vi "Inverse Kinematics.vi"() -> ()   [LabVIEW 2018]
uses:
  <vilib>/Platform/TimedLoop/XDataNode/timing_clust.ctl
  <vilib>/Platform/TimedLoop/XDataNode/nitl_modes.ctl
  <vilib>/Platform/TimedLoop/XDataNode/wakeup.ctl
  <extravilib>/ChannelInstances/Tag-bool/Read With Abort.vi
  <extravilib>/ChannelInstances/Tag-bool/Write With Abort.vi
  <extravilib>/ChannelInstances/Tag-bool/Instantiate.vi
  <extravilib>/ChannelInstances/Tag-bool/EndpointRead.vi
  <extravilib>/ChannelInstances/Tag-bool/Endpoint.vi
  <vilib>/Platform/TimedLoop/XDataNode/XDataNode.xnode
  <vilib>/Platform/TimedLoop/XDataNode/XDNodeRunTimeDep.lvlib
  <extravilib>/ChannelInstances/Tag-bool.lvlib
panel:
  out "Camera Image":T1(plugin-control)
  in  "Stop Button":bool
  out "Calibrated":bool
  out "Actual Joint \nCoordinates (rad)":dbl[](array[numeric])
  out "Joint Coordinates \nfrom Inv Kin (rad)":dbl[](array[numeric])
  in  "Task Coordinates for\nInv Kin (cm)":dbl[](array[numeric])=[3.81, 10.0]
  out "Motor angles (rad)":T2(graph)
  # "Mechatronic Systems Board"
  # "Inverse Kinematics"
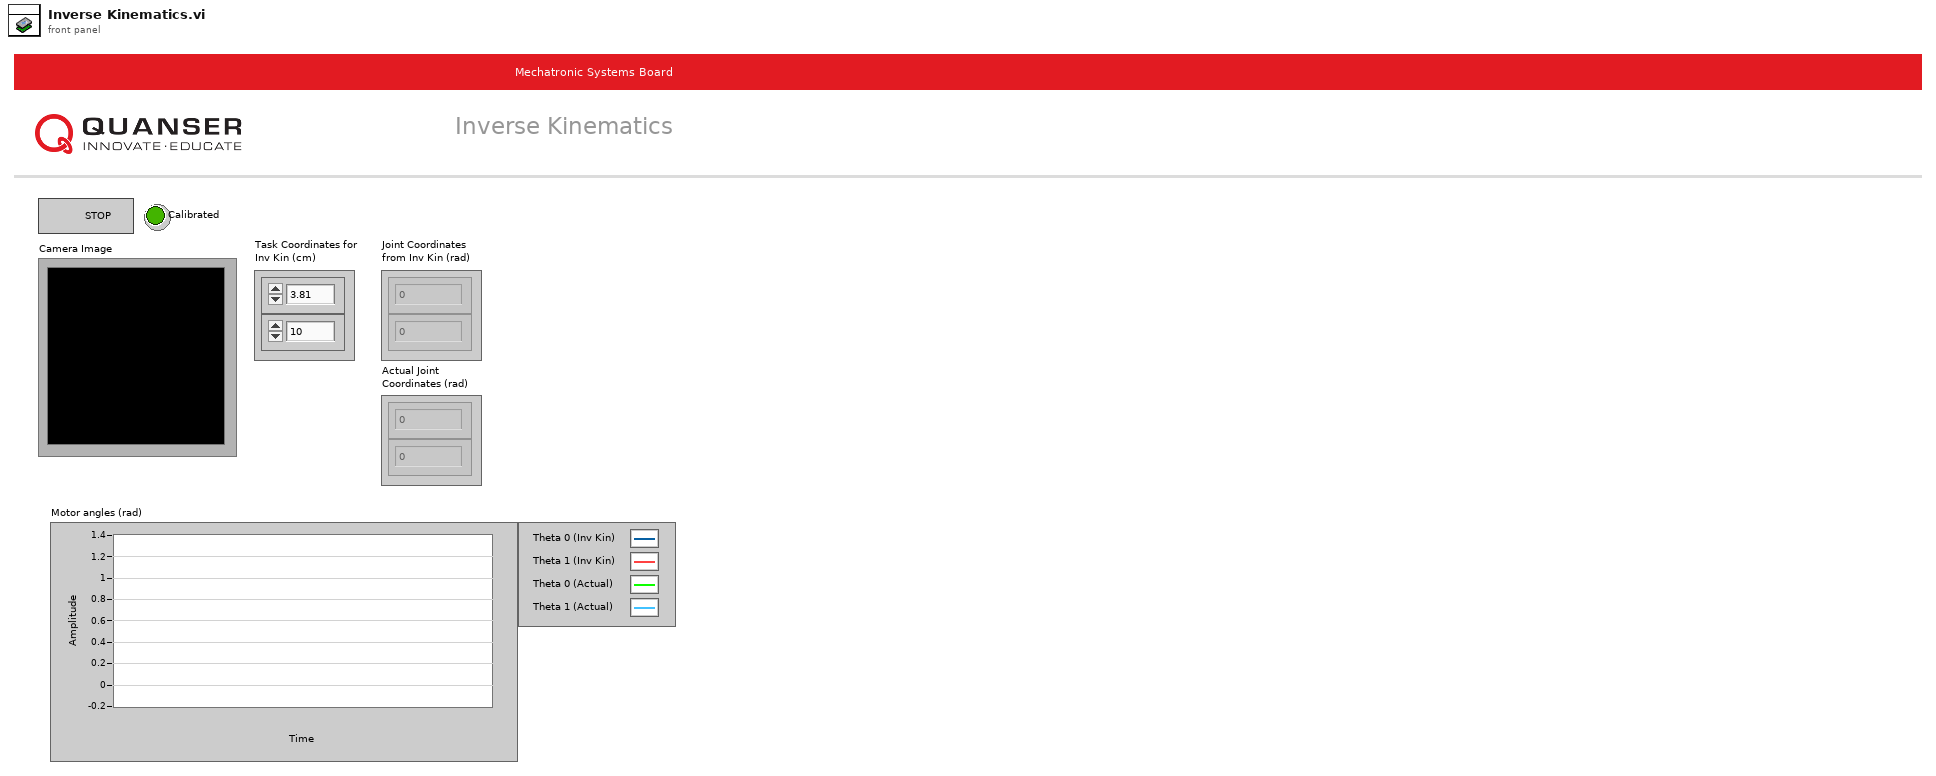
[diagram p1: front panel]
types:
  T1 = typedef "IMAQ Image.ctl" = refnum<image>
  T2 = cluster{dbl, dbl, "Numeric Control":dbl, "Numeric Control":dbl}
  T3 = typedef "QNET MS IO Cluster.ctl" = cluster{"Error":errorcluster, "Encoder Calibration Values":i32[], "Update Calibration":bool, "JPEG Resolutions":u16, "Raw Resolutions":u16, "Image Mode":enum16{"RAW RGB", "RAW Gray Scale", "JPEG"}, "FPGA Ref":refnum<k20>}
  T4 = typedef "XDNodeRunTimeDep.lvlib/timing_clust.ctl" = cluster{"Expected End [f-1]":u64, "Actual End [f-1]":u64, "Finished Late? [f-1]":bool, "Expected End [i-1]":u64, "Actual End [i-1]":u64, "Finished Late? [i-1]":bool, "Expected Start [i]":u64, "Actual Start [i]":u64, "Expected Start [f]":u64, "Actual Start [f]":u64, "Source Name":string, "Structure Name":string, "Period":i64, "Deadline":i64, "Offset":i64, "Start":i64, "Priority":i32, "Timeout":i32, "Mode":T5, "Wakeup Reason":T6, "Error":errorcluster, "Source Type":string, "Secondary Source Type":string, "Global End Time":u64, "Global Start Time":u64, "Frame Duration":u64, "Iteration Duration":u64, "Assigned CPU":i32, "I/O Scan Engine Mode":u32}
  T5 = typedef "XDNodeRunTimeDep.lvlib/nitl_modes.ctl" = enum32{"No Change", "Process missed periods, maintain original phase", "Discard missed periods, maintain original phase", "Process missed periods, ignore original phase", "Discard missed periods, ignore original phase"}
  T6 = typedef "XDNodeRunTimeDep.lvlib/wakeup.ctl" = enum32{"Normal", "Aborted", "Asynchronous wakeup", "Timing source error", "Timed loop error", "Timeout"}
  T7 = typedef "Tag-bool.lvlib/))Channel.ctl" = refnum<queue>
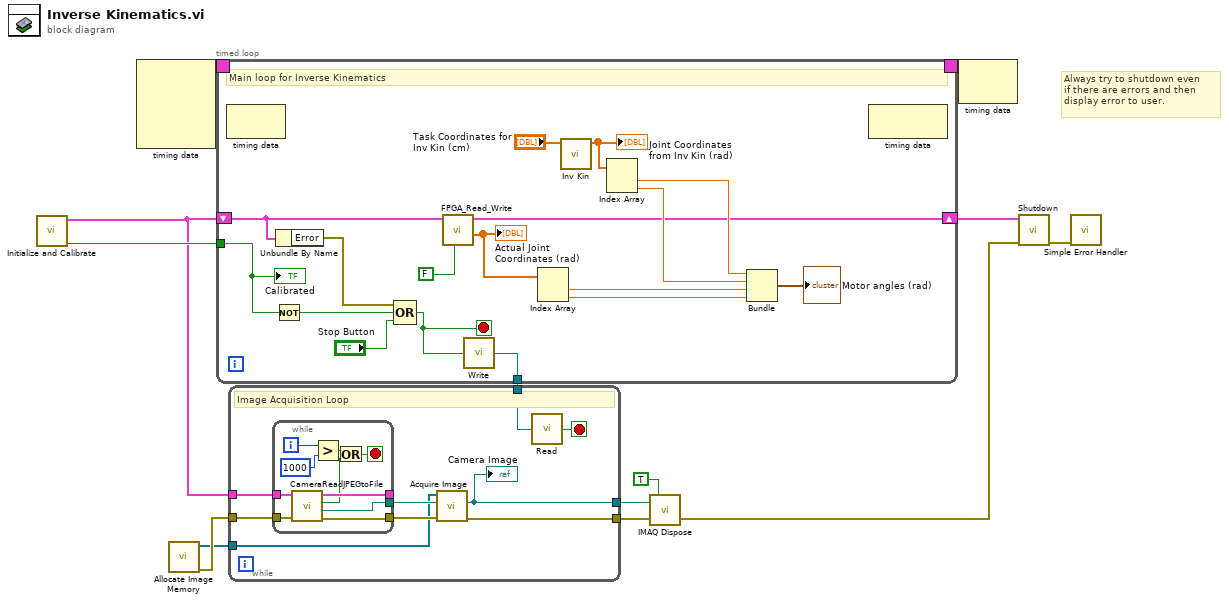
[diagram p0: block diagram]
diagram:
  # "Always try to shutdown even \nif there are errors and then \ndisplay error to user."
  n1 = call "Initialize and Calibrate.vi"() -> ("Calibrated"=w9:bool, "IO Cluster"=w8:T3)  [unwired: 10 in]
  n2 = node-c288() -> (w13:T4)  [unwired: 4 in]
  n3 = call "Allocate Image Memory.vi"() -> ("error out"=w7:errorcluster, "Acquisition Memory"=w6:T1[])  [unwired: 6 in, 4 out]
  n4 = timed-loop {
    timing: w13 -> [_]
    timing-out: [_] -> w12
    tunnel: w9 -> [w17]
    shift-right: [w21] -> w10
    shift-left: w8 -> [w20]
    tunnel: [w14] -> w1
    stop <- w15 stop-if-true
    # "Main loop for Inverse Kinematics"
    n5 = node-c288() -> ()  [unwired: 1 in, 1 out]
    n6 = Not(x=w17) -> (.not. x?=w16:bool)
    n7 = Unbundle By Name(w20) -> ("Error"=w19:errorcluster)
    n8 = Compound Arithmetic op=OR(w19, w16, "Stop Button") -> (w15:bool)
    n9 = call "FPGA_Read_Write.vi"("Motors enabled?"=FALSE ("Motors Enabled"), "IO Cluster In"=w20) -> ("Joint Coordinates (rad)"=w22:dbl[], "IO Cluster Out"=w21:T3)  [unwired: 6 in, 2 out]
    "Actual Joint \nCoordinates (rad)" <- w22
    n10 = call <extravilib>:"Write.vi"("element"=w15) -> ("channel"=w14:T7)  [unwired: 1 out]
    n11 = Index Array(array=w22) -> (element #1=w27:dbl, element #2=w25:dbl)  [unwired: 2 in]
    n12 = call "Inv Kin.vi"("Task Coordinates (cm)"="Task Coordinates for\nInv Kin (cm)") -> ("Joint Coordinates (rad)"=w30:dbl[])  [unwired: 10 in]
    "Joint Coordinates \nfrom Inv Kin (rad)" <- w30
    n13 = Index Array ("Index Array 2")(array=w30) -> (element #1=w24:dbl, element #2=w26:dbl)  [unwired: 2 in]
    n14 = Bundle(w24, w26, "Numeric Control"=w27, "Numeric Control"=w25) -> (→"Motor angles (rad)":T2)  [unwired: 1 in]
    n15 = node-c288() -> ()  [unwired: 1 in, 1 out]
    "Calibrated" <- w17
  }
  n16 = while {
    tunnel: w8 -> [w39]
    tunnel: w7 -> [w38]
    tunnel: w6 -> [w37]
    tunnel: [w36] -> w3
    tunnel: [w35] -> w4
    tunnel: w1 -> [w34]
    stop <- w33 stop-if-true
    # "Image Acquisition Loop"
    n17 = while {
      tunnel: [w47] -> w40
      tunnel: w39 -> [w51]
      tunnel: [w50] -> _
      tunnel: w38 -> [w48]
      tunnel: [w49] -> w41
      i -> [w43]
      stop <- w46 stop-if-true
      n18 = call "CameraReadJPEGtoFile.vi"("error in"=w48, "IO Cluster In"=w51) -> ("Error Out"=w49:errorcluster, "Image File"=w47:path, "New Image Data"=w42:bool, "IO Cluster Out"=w50:T3)  [unwired: 6 in]
      n19 = Greater?(x=w43, y=1000) -> (0:w45:bool)
      n20 = Or(x=w45, y=w42) -> (x .or. y?=w46:bool)
    }
    n21 = call "Acquire Image.vi"("Error In"=w41, "File Path"=w40, "Acquisition Memory"=w37) -> ("Error Out"=w36:errorcluster, "HSL Image"=w35:T1)  [unwired: 4 in, 3 out]
    "Camera Image" <- w35
    n22 = call <extravilib>:"Read.vi"("channel"=w34) -> ("element"=w33:bool)  [unwired: 1 in, 1 out]
  }
  n23 = call "IMAQ Dispose"("All Images? (No)"=TRUE, "Image"=w4, "error in (no error)"=w3) -> ("error out"=w2:errorcluster)  [unwired: 3 in]
  n24 = node-c288(w12) -> ()  [unwired: 1 out]
  n25 = call "Shutdown.vi"("Image Processing Loop"=w2, "IO Cluster In"=w10) -> ("Error"=w11:errorcluster)  [unwired: 9 in]
  n26 = call <vilib>:"Simple Error Handler.vi"("error in (no error)"=w11) -> ()  [unwired: 4 in, 5 out]
